vi "Button Pressed Event.vi"(8 "error in (no error)":errorcluster, 9 "Data":variant, 10 "CtlRef":refnum<vi>, 11 "uService Template in":refnum<class "Father of all uServices.lvclass">) -> (0 "error out":errorcluster, 3 "uService Template out":refnum<class "Father of all uServices.lvclass">)   [LabVIEW 2026, in "TALOS.lvlib" / "Father of all uServices.lvlib" / "Father of all uServices.lvclass"]
uses:
  Father of all uServices.lvclass
  Event Handler Items.ctl
  Ancestor/Ancestor/Ancestor.lvclass/Ancestor.ctl
  Support VIs/Generate Error.vi
  FGV/Error Memory/Get Error Description.vi
  Support VIs/Get PC name.vi
  Ancestor/Ancestor/Read ID.vi
  Support VIs/Get Class Name.vi
  <vilib>/Utility/error.llb/Clear Errors.vi
  FGV/Error Memory/Error Memory Core.vi
  <vilib>/AdvancedString/Delimited String to 1D String Array.vi
  <vilib>/AdvancedString/Delimited String to 1D String Array (string).vi
  Support VIs/Circus Root Path.vi
  FGV/Error Memory/Error Crt Lvl checker.vi
  FGV/Error Memory/Error Memory Core.vi/40c8088d-b597-4017-91af-faa98e00292e.vi
  FGV/Error Memory/Error Memory Core.vi/d4a3ab98-063c-4e44-b43d-fbdcfe6c2be2.vi
  Support VIs/Global Memory.vi
  <vilib>/Utility/LVClass/Get LV Class Name.vi
  Support VIs/Is in Packed Library.vi
  Support VIs/TALOS Root path.vi
  Support VIs/Read CSV worksheet.vi
  Support VIs/Global Constants.vi
  <vilib>/Utility/error.llb/General Error Handler.vi
  Support VIs/Error Log.vi
  Ancestor/Ancestor/Ancestor.lvclass
  <vilib>/Comparison/Equal/Equal Functor/Equal Functor.lvclass
  TALOS.lvlib
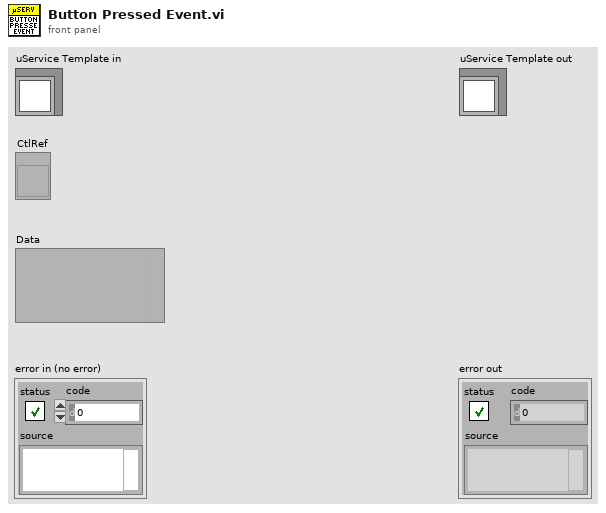
[diagram p1: front panel]
types:
  T1 = typedef "TALOS.lvlib/Father of all uServices.lvlib/Father of all uServices.lvclass/Event Handler Items.ctl" = enum16{"Button Pressed", "Message", "Ready to launch?", "Safe Mode", "Start RUN", "Stop RUN"}
  T2 = cluster{"Event Item":T1, "Event Item Name":string, "Event Data":variant}
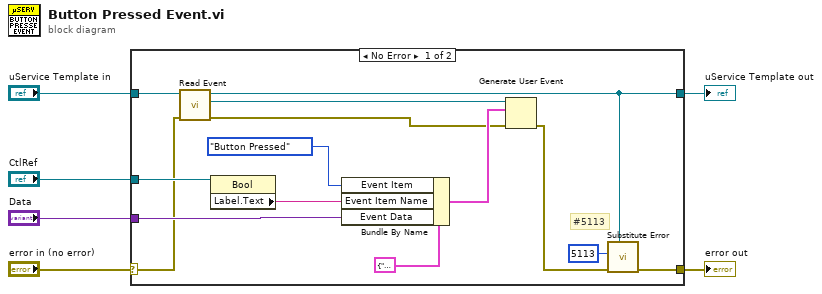
[diagram p0: block diagram]
diagram:
  n1 = case shown="No Error" "error in (no error)" {
    selector: "error in (no error)" -> [w13 w22]
    tunnel: [w9 w22] -> w5
    tunnel: [w8 w21] -> w3
    tunnel: "uService Template in" -> [w12 w21]
    tunnel: "CtlRef" -> [w15 _]
    tunnel: "Data" -> [w14 _]
    frame No Error {
      # "#5113"
      n2 = call-dynamic "Read Event.vi"("error in (no error)"=w13, "uService Template in"=w12) -> ("error out"=w11:errorcluster, "Event"=w20:refnum<user-event>, "uService Template out"=w8:refnum<class "Father of all uServices.lvclass">)  [unwired: 7 in]
      n3 = property class="Bool"(reference=w15) -> ("Label.Text"=w17:string)  [unwired: 1 in, 2 out]
      n4 = Bundle By Name(cluster=T2 {"Event Item"=enum."Button Pressed", "Event Item Name"="", "Event Data"=variant} ("event data"), "Event Item"=Event_Handler_Items."Button Pressed", "Event Item Name"=w17, "Event Data"=w14) -> (w19:T2)
      n5 = Generate User Event(user event=w20, event data cluster=w19, error in=w11) -> (error out=w10:errorcluster)  [unwired: 1 in, 1 out]
      n6 = call "Substitute Error.vi"("LabVIEW Object"=w8, "error in (no error)"=w10, "Error Code"=5113) -> ("error out"=w9:errorcluster)  [unwired: 8 in]
    }
    frame Error {
    }
  }
  "error out" <- w5
  "uService Template out" <- w3
